vi "Deploy Ramps.vi"(10 "Deploy":bool, 11 "refnum name":string="LeftRamp") -> (3 "Output":bool)   [LabVIEW 2017]
uses:
  <vilib>/Rock Robotics/WPI/Solenoid/WPI_SolenoidValue.ctl
  <vilib>/Rock Robotics/WPI/Solenoid/WPI_SolenoidSetEnum.vi
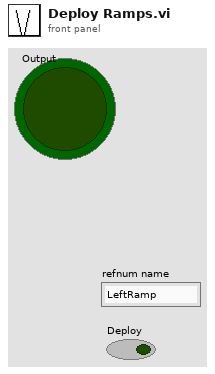
[diagram p1: front panel]
types:
  T1 = typedef "WPI_SolenoidValue.ctl" = enum16{"Off", "On", "Forward", "Reverse"}
  T2 = typedef "WPI_SolenoidDevRef.ctl" = cluster{"DevStatus":errorcluster, "Pneumatics Control Module":u8, "Forward Solenoid Channel":T3, "Reverse Solenoid Channel":T3}
  T3 = typedef "WPI_SolenoidChannel.ctl" = enum8{"Solenoid 0", "Solenoid 1", "Solenoid 2", "Solenoid 3", "Solenoid 4", "Solenoid 5", "Solenoid 6", "Solenoid 7", "Invalid"}
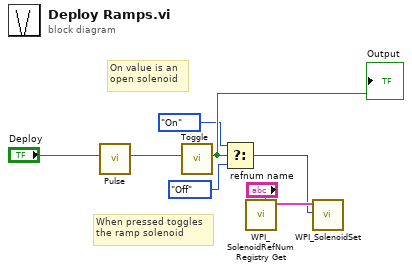
[diagram p0: block diagram]
diagram:
  # "On value is an \nopen solenoid"
  # "When pressed toggles\nthe ramp solenoid"
  n1 = call "Pulse.vi"("Input"="Deploy") -> ("Output"=w1:bool)  [unwired: 10 in]
  n2 = call "Toggle.vi"("Input"=w1) -> ("Output"=w6:bool)  [unwired: 10 in]
  "Output" <- w6
  n3 = Select(t=WPI_SolenoidValue."On" ("Value"), s=w6, f=WPI_SolenoidValue."Off" ("Value")) -> (s? t:f=w3:T1)
  n4 = call <vilib>:"WPI_SolenoidRefNum Registry Get.vi"("refnum name"="refnum name") -> ("SolenoidDevRef"=w8:T2)  [unwired: 9 in, 1 out]
  n5 = call-poly <vilib>:"WPI_SolenoidSet.vi"("Value"=w3, "SolenoidDevRef"=w8) -> ()  [unwired: 8 in, 2 out]
